vi "Laplace PDF.vi"(9 "b":dbl=1.0, 10 "a":dbl=1.0, 11 "x":dbl) -> (0 "error":i32, 3 "pdf(x)":dbl=0.18393972058572117)   [LabVIEW 2017, in "NI_Gmath.lvlib"]
doc: "Computes the continuous probability density function (PDF) of various distributions. You must manually select the polymorphic instance to use."
uses:
  NI_Gmath.lvlib
  st_error_code.ctl
panel:
  # "Laplace PDF"
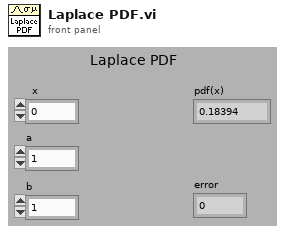
[diagram p1: front panel]
types:
  T1 = typedef "NI_Gmath.lvlib/st_error_code.ctl" = i32
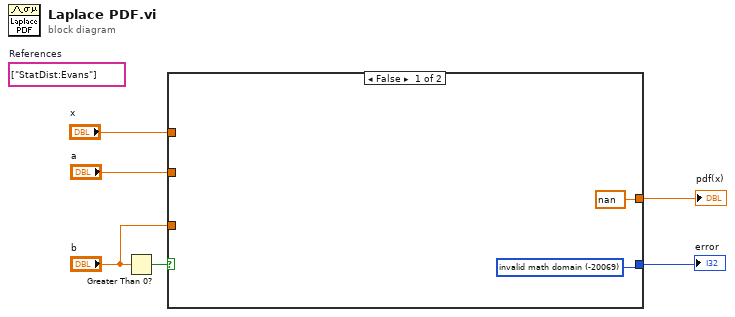
[diagram p0: block diagram]
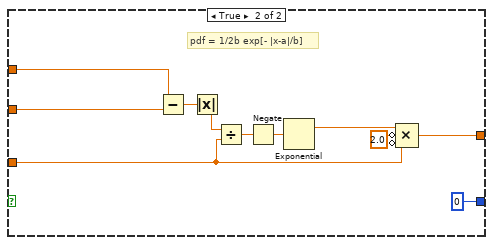
[diagram p2: hidden frame]
diagram:
  (unwired) string[] ["StatDist:Evans"]  # References
  n1 = Greater Than 0?(x="b") -> (x > 0?=w2:bool)
  n2 = case shown="False" w2 {
    tunnel: "b" -> [_ w15]
    tunnel: [w7 0 ("invalid math domain")] -> w6
    tunnel: [nan w14] -> w5
    tunnel: "x" -> [_ w18]
    tunnel: "a" -> [_ w17]
    frame False {
      w7 = T1 -20069 items=["invalid math domain"=-20069, "Fourier interpolation size m >= n"=-20070, "empty array"=-20003] ("stat interp error code")
    }
    frame True {
      # "pdf = 1/2b exp[- |x-a|/b]"
      n3 = Subtract(x=w18, y=w17) -> (x-y=w16:dbl)
      n4 = Absolute Value(x=w16) -> (abs(x)=w12:dbl)
      n5 = Divide(x=w12, y=w15) -> (x/y=w13:dbl)
      n6 = Negate(x=w13) -> (-x=w11:dbl)
      n7 = Exponential(1:w11) -> (0:w10:dbl)
      n8 = Compound Arithmetic op=MULTIPLY(w10, invert 2.0 ("value"), invert w15) -> (w14:dbl)
    }
  }
  "pdf(x)" <- w5
  "error" <- w6
